vi "Read Data.vi"(8 "error in (no error)":errorcluster, 11 "Log Message in":refnum<class "Check Size Message.lvclass">) -> (0 "error out":errorcluster, 2 "Data":T1[](array[typedef]), 3 "Log Message out":refnum<class "Check Size Message.lvclass">)   [LabVIEW 2020, in "AIM ARINC 664 Engine.lvlib" / "Implementation.lvlib" / "Frame Logging.lvlib" / "Check Size Message.lvclass"]
uses:
  Check Size Message.lvclass
  Frame.ctl
  Check Size Message.lvclass/Check Size Message.ctl
  Implementation.lvlib
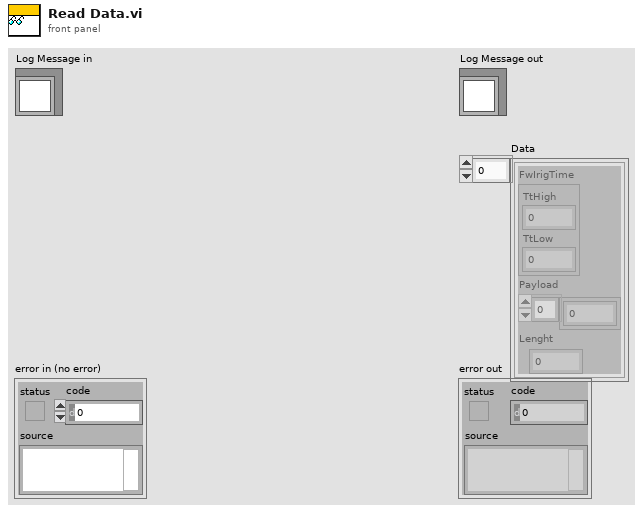
[diagram p1: front panel]
types:
  T1 = typedef "AIM ARINC 664 Engine.lvlib/Implementation.lvlib/Frame.ctl" = cluster{"FwIrigTime":cluster{"TtHigh":u32, "TtLow":u32}, "Payload":u8[], "Lenght":u32}
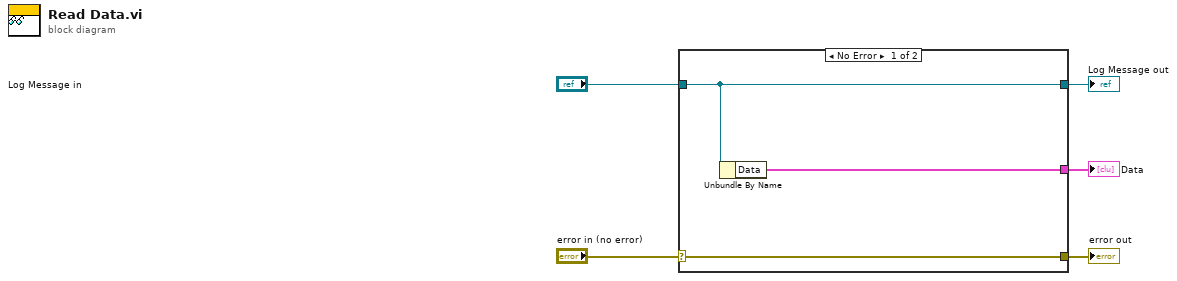
[diagram p0: block diagram]
diagram:
  n1 = case shown="No Error" "error in (no error)" {
    selector: "error in (no error)" -> [w8 w9]
    tunnel: [w8 w9] -> w4
    tunnel: [w7 w10] -> w2
    tunnel: "Log Message in" -> [w7 w10]
    tunnel: [w6 _] -> w1
    frame No Error {
      n2 = Unbundle By Name(w7) -> ("Data"=w6:T1[])
    }
    frame Error {
    }
  }
  "error out" <- w4
  "Log Message out" <- w2
  "Data" <- w1
